vi "Simulate_kernal.vi"() -> ()   [LabVIEW 2011]
uses:
  Globals/Meas_global.vi
  <vilib>/Analysis/NI_AALBase.lvlib
panel:
  out "Waveform Graph":dbl[][](graph)
  in  "Random?":bool
  in  "Average Value":dbl
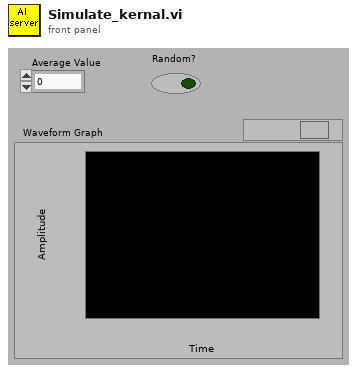
[diagram p1: front panel]
types:
  T1 = typedef "Ch_and_Spans.ctl" = cluster{"high limit (10V)":sgl, "low limit (-10V)":sgl, "Ch No":i16, "Var name":string, "Use Latest Calib":bool}
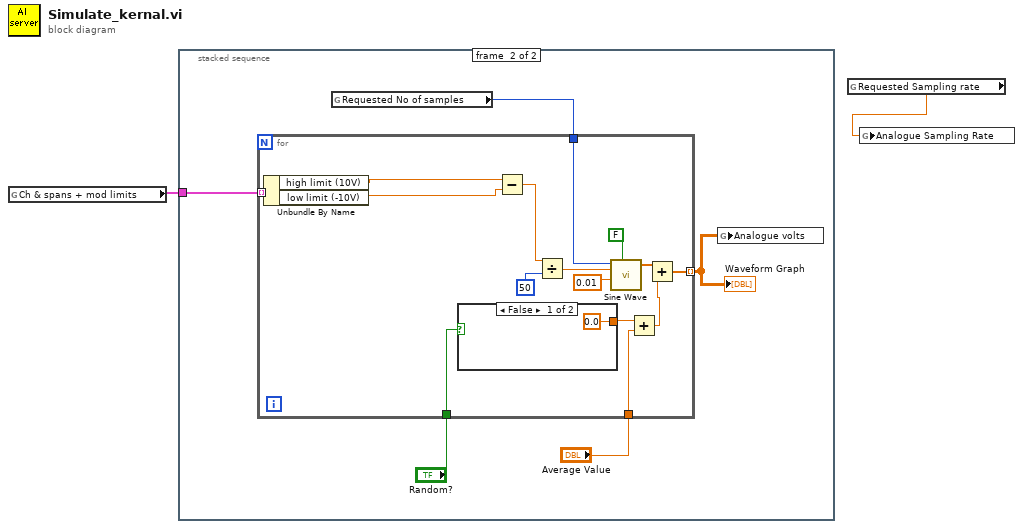
[diagram p0: block diagram]
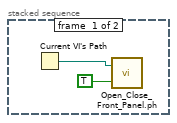
[diagram p2: hidden frame]
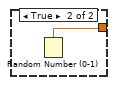
[diagram p3: hidden frame]
diagram:
  n1 = global read "Meas_global.vi" "Ch & spans + mod limits"() -> (w2:T1[])
  n2 = stacked-sequence {
    tunnel: w2 -> [_ w9]
    frame #0 {
      n3 = Current VI's Path() -> (path=w4:path)
      n4 = call "Open_Close_Front_Panel.ph.vi"("Front Panel Window:Open"=TRUE, "VI path"=w4) -> ()  [unwired: 2 out]
    }
    frame #1 {
      n5 = global read "Meas_global.vi" "Requested No of samples"() -> (w6:i32)
      n6 = for {
        tunnel: [w16] -> w5 mode=indexing
        tunnel: w6 -> [w17]
        tunnel: w9 -> [w19] mode=indexing
        tunnel: "Random?" -> [w18]
        tunnel: "Average Value" -> [w12]
        n7 = Unbundle By Name(w19) -> ("high limit (10V)"=w11:sgl, "low limit (-10V)"=w10:sgl)
        n8 = case shown="False" w18 {
          tunnel: [0.0 ("number: 0 to 1") w26] -> w14
          frame False {
          }
          frame True {
            n9 = Random Number (0-1)() -> (number: 0 to 1=w26:dbl)
          }
        }
        n10 = Subtract(x=w11, y=w10) -> (x-y=w15:sgl)
        n11 = Divide(x=w15, y=50) -> (x/y=w21:sgl)
        n12 = call <vilib>:"Sine Wave.vi"("samples"=w17, "amplitude"=w21, "frequency"=0.01 ("f"), "reset phase"=FALSE) -> ("sine wave"=w23:dbl[])  [unwired: 1 in, 2 out]
        n13 = Add(x=w14, y=w12) -> (x+y=w13:dbl)
        n14 = Add(x=w23, y=w13) -> (x+y=w16:dbl[])
      }
      "Waveform Graph" <- w5
      n15 = global write "Meas_global.vi" "Analogue volts"(w5) -> ()
    }
  }
  n16 = global read "Meas_global.vi" "Requested Sampling rate"() -> (w1:dbl)
  n17 = global write "Meas_global.vi" "Analogue Sampling Rate"(w1) -> ()
